vi "RemoveChildFromNode.vi"(8 "error in":errorcluster, 10 "removed child":T1, 11 "CEF_Node in":refnum<class "CEF_Node.lvclass">) -> (0 "error out":errorcluster, 3 "CEF_Node out":refnum<class "CEF_Node.lvclass">)   [LabVIEW 2023, in "CEF.lvlib" / "CEF_Node.lvclass"]
doc: "Copyright 2017 National Instruments Corporation\n\nLicensed under the Apache License, Version 2.0 (the \"License\"); you may not use this file except in compliance with the License. You may obtain a copy of the License at http://www.apache.org/licenses/LICENSE-2.0\nUnless required by applicable law or agreed to in writing, software distributed under the License is distributed on an \"AS IS\" BASIS, WITHOUT WARRANTIES OR CONDITIONS OF ANY KIND, either express or implied. See the License for the specific language governing permissions and limitations under the License."
uses:
  CEF_Node.lvclass
  NodeRef.ctl
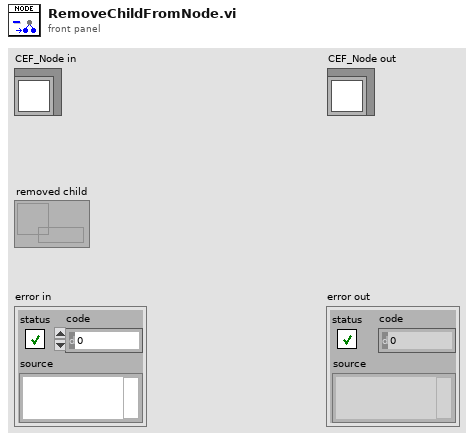
[diagram p1: front panel]
types:
  T1 = typedef "CEF.lvlib/CEF_Node.lvclass/NodeRef.ctl" = refnum<data-value>
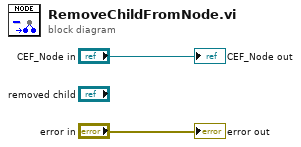
[diagram p0: block diagram]
diagram:
  "error out" <- "error in"
  "CEF_Node out" <- "CEF_Node in"
